vi "CreateOrganizedLogFolderStructure.vi"(8 "Error In":errorcluster, 10 "Time Stamp":timestamp, 11 "Base Log Path":path) -> (0 "Error Out":errorcluster, 3 "Organized Log Path":path)   [LabVIEW 2012]
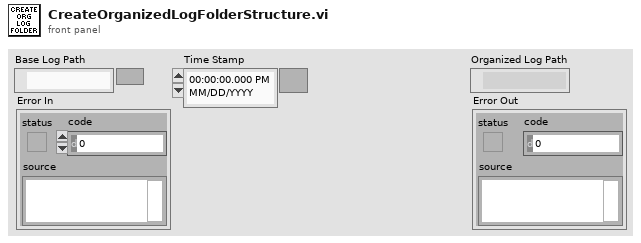
[diagram p1: front panel]
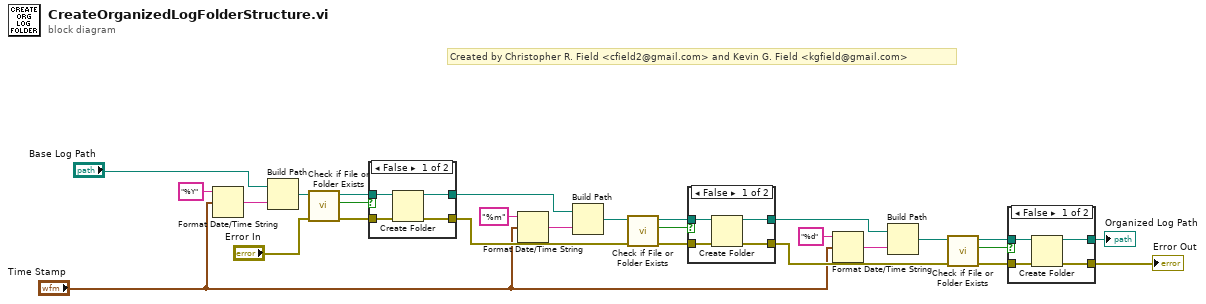
[diagram p0: block diagram]
diagram:
  # "Created by Christopher R. Field <cfield2@gmail.com> and Kevin G. Field <kgfield@gmail.com>"
  n1 = Format Date/Time String(time format string (%c)="%Y", seconds (now)="Time Stamp") -> (date/time string=w26:string)  [unwired: 1 in]
  n2 = Build Path(base path="Base Log Path", name or relative path=w26) -> (appended path=w20:path)
  n3 = call <vilib>:"Check if File or Folder Exists.vi"("error in (no error)"="Error In", "path"=w20) -> ("error out"=w17:errorcluster, "file or folder exists?"=w19:bool, "dup path"=w18:path)  [unwired: 7 in]
  n4 = case shown="False" w19 {
    tunnel: w18 -> [w31 w33]
    tunnel: w17 -> [w30 w32]
    tunnel: [w29 w33] -> w16
    tunnel: [w28 w32] -> w14
    frame False {
      n5 = Create Folder(path (use dialog)=w31, error in=w30) -> (created path=w29:path, error out=w28:errorcluster)  [unwired: 1 in, 1 out]
    }
    frame True {
    }
  }
  n6 = Format Date/Time String(time format string (%c)="%m", seconds (now)="Time Stamp") -> (date/time string=w24:string)  [unwired: 1 in]
  n7 = Build Path(base path=w16, name or relative path=w24) -> (appended path=w15:path)
  n8 = call <vilib>:"Check if File or Folder Exists.vi"("error in (no error)"=w14, "path"=w15) -> ("error out"=w12:errorcluster, "file or folder exists?"=w11:bool, "dup path"=w13:path)  [unwired: 7 in]
  n9 = case shown="False" w11 {
    tunnel: w13 -> [w37 w39]
    tunnel: w12 -> [w36 w38]
    tunnel: [w35 w39] -> w7
    tunnel: [w34 w38] -> w5
    frame False {
      n10 = Create Folder(path (use dialog)=w37, error in=w36) -> (created path=w35:path, error out=w34:errorcluster)  [unwired: 1 in, 1 out]
    }
    frame True {
    }
  }
  n11 = Format Date/Time String(time format string (%c)="%d", seconds (now)="Time Stamp") -> (date/time string=w22:string)  [unwired: 1 in]
  n12 = Build Path(base path=w7, name or relative path=w22) -> (appended path=w6:path)
  n13 = call <vilib>:"Check if File or Folder Exists.vi"("error in (no error)"=w5, "path"=w6) -> ("error out"=w9:errorcluster, "file or folder exists?"=w8:bool, "dup path"=w10:path)  [unwired: 7 in]
  n14 = case shown="False" w8 {
    tunnel: w10 -> [w43 w45]
    tunnel: w9 -> [w42 w44]
    tunnel: [w41 w45] -> w4
    tunnel: [w40 w44] -> w3
    frame False {
      n15 = Create Folder(path (use dialog)=w43, error in=w42) -> (created path=w41:path, error out=w40:errorcluster)  [unwired: 1 in, 1 out]
    }
    frame True {
    }
  }
  "Organized Log Path" <- w4
  "Error Out" <- w3
